vi "dfd_Group Delay Create Specs.vi"(6 "fs [Hz]":dbl=1.0 format="%.2f", 8 "error in (no error)":errorcluster, 10 "freq range":cluster{"f lo":dbl, "f hi":dbl}[](array[cluster]), 11 "filter in":T1={"mSRate_Fs"=1.0, "mSRate_Version"="1.0", "mSRate_Comments"="", "mSRate_OrgCoef"={"type"=enum."Undefined", "gain"=1.0, "coef a (k)"=[], "coef b (v)"=[]}, "mSRate_CurCoef"={"type"=enum."Undefined", "gain"=1.0, "coef a (k)"=[], "coef b (v)"=[]}, "mSRate_Quantized?"=FALSE, "mSRate_QCoef"={"type"=enum."Undefined", "gain"=1.0, "coef a (k)"=[], "coef b (v)"=[]}, "mSRate_QSettings"=[], "mSRate_Order"=0, "mSRate_Scaling"={"mSRate_ScaleByPowerOf2?"=FALSE, "mSRate_ScaleType"=enum."No Norm"}} {"mSRate_QSettings"."source" items=["Coef a/k"=0, "Coef b/v"=7, "Input"=1, "Output"=2, "Multiplicand"=3, "Product"=4, "Sum"=5, "Delay"=6, "Gain"=8]}) -> (0 "error out":errorcluster, 2 "band specs":T7[](array[typedef]) {"subband specs"."weight" format="%.2f"}, 3 "filter out":T1={"mSRate_Fs"=1.0, "mSRate_Version"="1.0", "mSRate_Comments"="", "mSRate_OrgCoef"={"type"=enum."Undefined", "gain"=1.0, "coef a (k)"=[], "coef b (v)"=[]}, "mSRate_CurCoef"={"type"=enum."Undefined", "gain"=1.0, "coef a (k)"=[], "coef b (v)"=[]}, "mSRate_Quantized?"=FALSE, "mSRate_QCoef"={"type"=enum."Undefined", "gain"=1.0, "coef a (k)"=[], "coef b (v)"=[]}, "mSRate_QSettings"=[], "mSRate_Order"=0, "mSRate_Scaling"={"mSRate_ScaleByPowerOf2?"=FALSE, "mSRate_ScaleType"=enum."No Norm"}} {"mSRate_QSettings"."source" items=["Coef a/k"=0, "Coef b/v"=7, "Input"=1, "Output"=2, "Multiplicand"=3, "Product"=4, "Sum"=5, "Delay"=6, "Gain"=8]})   [LabVIEW 2017, in "NI_DigFilter_Design.lvlib"]
uses:
  <vilib>/addons/Digital Filter Design/NI_DigFilter_Design.lvlib
  <vilib>/addons/Digital Filter Design/_GroupDelay.llb/dfd_Group Delay_Band Spec.ctl
  <vilib>/addons/Digital Filter Design/_Objects.llb/DFD Filter Obj.ctl
  <vilib>/addons/Digital Filter Design/_Objects.llb/DFD Filter Coef.ctl
  <vilib>/addons/Digital Filter Design/_Objects.llb/DFD Filter Structure Type Selector.ctl
  <vilib>/addons/Digital Filter Design/_Objects.llb/dfd_Internal Quantization Settings.ctl
  <vilib>/addons/Digital Filter Design/_Objects.llb/dfd_Internal Quantization Srcs.ctl
  <vilib>/addons/Digital Filter Design/_Objects.llb/DFD Coef Norm Type.ctl
  <vilib>/Analysis/1siggen.llb/Ramp Pattern by Samples.vi
  <vilib>/addons/Digital Filter Design/NI_DigFilterLicensed.lvlib
  <vilib>/Analysis/NI_AALBase.lvlib
panel:
  in  "?":T7={"subband specs"=[{"freq"=0.0, "group delay"=1.0, "weight"=1.0}, {"freq"=0.2, "group delay"=1.0, "weight"=1.0}]} {"subband specs"."weight" format="%.2f"}
  # "freq"
  # "group delay"
  # "weight"
  # "freq"
  # "group delay"
  # "weight"
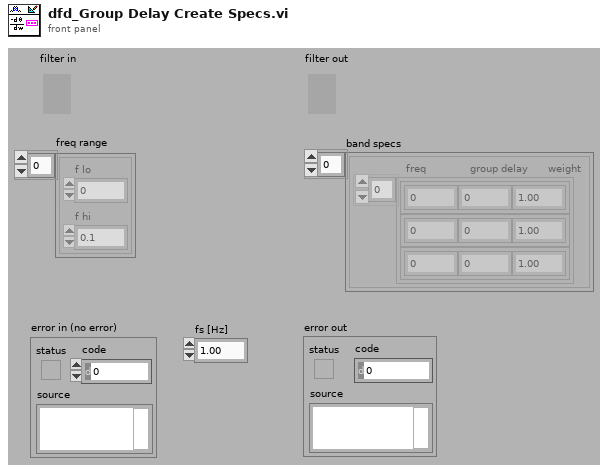
[diagram p1: front panel]
types:
  T1 = typedef "NI_DigFilterLicensed.lvlib/DFD Filter Obj.ctl" = cluster{"mSRate_Fs":dbl, "mSRate_Version":string, "mSRate_Comments":string, "mSRate_OrgCoef":T2, "mSRate_CurCoef":T2, "mSRate_Quantized?":bool, "mSRate_QCoef":T2, "mSRate_QSettings":T4[], "mSRate_Order":i32, "mSRate_Scaling":cluster{"mSRate_ScaleByPowerOf2?":bool, "mSRate_ScaleType":T6}}
  T2 = typedef "NI_DigFilterLicensed.lvlib/DFD Filter Coef.ctl" = cluster{"type":T3, "gain":dbl, "coef a (k)":dbl[], "coef b (v)":dbl[]}
  T3 = typedef "NI_DigFilterLicensed.lvlib/DFD Filter Structure Type Selector.ctl" = enum16{"Undefined", "FIR Direct Form", "FIR Direct Form Transposed", "FIR Symmetric", "FIR Antisymmetric", "IIR Direct Form I", "IIR Direct Form I Transposed", "IIR Direct Form II", "IIR Direct Form II Transposed", "IIR Cascaded Second Order Sections Form I", "IIR Cascaded Second Order Sections Form I Transposed", "IIR Cascaded Second Order Sections Form II", "IIR Cascaded Second Order Sections Form II Transposed", "Lattice Allpass (basic sections)", "Lattice Allpass (one multiplier sections)", "Lattice Allpass (normalized sections)", "Lattice AR (basic sections)", "Lattice AR (one multiplier sections)", "Lattice AR (normalized sections)", "Lattice MA (minimum phase)", "Lattice MA (maximum phase)", "Lattice ARMA (basic sections)", "Lattice ARMA (one multiplier sections)", "Lattice ARMA (normalized sections)"}
  T4 = typedef "NI_DigFilterLicensed.lvlib/dfd_Internal Quantization Settings.ctl" = cluster{"source":T5, "wl":i16, "iwl":i16, "overflow mode":enum16{"Saturation", "Wrap"}, "rounding mode":enum16{"Nearest", "Truncation"}, "signed?":bool}
  T5 = typedef "NI_DigFilterLicensed.lvlib/dfd_Internal Quantization Srcs.ctl" = u16
  T6 = typedef "NI_DigFilterLicensed.lvlib/DFD Coef Norm Type.ctl" = enum16{"No Norm", "Time Domain 1-Norm", "Time Domain 2-Norm", "Time Domain Inf-Norm"}
  T7 = typedef "NI_DigFilterLicensed.lvlib/dfd_Group Delay_Band Spec.ctl" = cluster{"subband specs":cluster{"freq":dbl, "group delay":dbl, "weight":dbl}[]}
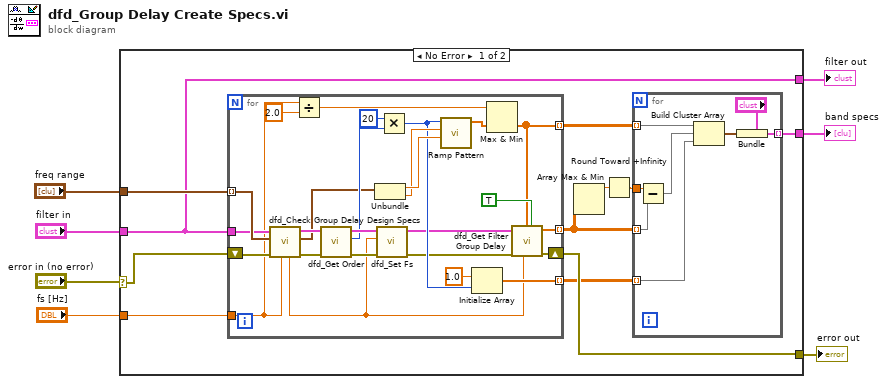
[diagram p0: block diagram]
diagram:
  n1 = case shown="No Error" "error in (no error)" {
    selector: "error in (no error)" -> [w17 w54]
    tunnel: "freq range" -> [w15 _]
    tunnel: "fs [Hz]" -> [w16 _]
    tunnel: "filter in" -> [w13 w53]
    tunnel: [w18 w54] -> w3
    tunnel: [w13 w53] -> w2
    tunnel: [w14 _] -> w1
    frame No Error {
      n2 = for {
        tunnel: w16 -> [w29]
        tunnel: w15 -> [w50] mode=indexing
        tunnel: w13 -> [w49]
        tunnel: [w30] -> w12 mode=indexing
        tunnel: [w47] -> w11 mode=indexing
        tunnel: [w44] -> w10 mode=indexing
        shift-right: [w52] -> w18
        shift-left: w17 -> [w51]
        n3 = call <vilib>:"dfd_Check Group Delay Design Specs.vi"("fs [Hz]"=w29, "error in (no error)"=w51, "freq range"=w50, "filter in"=w49) -> ("error IO"=w35:errorcluster, "dup freq range"=w32:cluster{"f lo":dbl, "f hi":dbl}, "dup filter in"=w33:T1, "dup fs [Hz]"=w34:dbl)  [unwired: 4 out]
        n4 = Divide(x=w29, y=2.0) -> (x/y=w27:dbl)
        n5 = call <vilib>:"dfd_Get Order.vi"("error in (no error)"=w35, "filter in"=w33) -> ("error out"=w41:errorcluster, "order"=w39:i32, "filter out"=w42:T1)  [unwired: 7 out]
        n6 = Unbundle(w32) -> ("f lo"=w46:dbl, "f hi"=w45:dbl)
        n7 = call <vilib>:"dfd_Set Fs.vi"("error in (no error)"=w41, "fs [Hz]"=w34, "filter in"=w42) -> ("error out"=w37:errorcluster, "filter out"=w36:T1)  [unwired: 7 out]
        n8 = Multiply(x=20, y=w39) -> (x*y=w38:i32)
        n9 = call-poly <vilib>:"Ramp Pattern.vi"("start"=w46, "end"=w45, "samples"=w38) -> ("Ramp Pattern"=w31:dbl[])  [unwired: 7 in, 1 out]
        n10 = Initialize Array(1.0 ("element"), w38) -> (w47:dbl[])
        n11 = Max & Min(x=w27, y=w31) -> (min(x,y)=w30:dbl[])  [unwired: 1 out]
        n12 = call <vilib>:"dfd_Get Filter Group Delay.vi"("output option\n(T: FLP)"=TRUE ("output option\n(T: FLP)"), "fs [Hz]"=w34, "freq points [Hz]"=w30, "error in (no error)"=w37, "filter in"=w36) -> ("error out"=w52:errorcluster, "group delay"=w44:dbl[])  [unwired: 5 out]
      }
      n13 = Array Max & Min(array=w10) -> (max value=w9:dbl)  [unwired: 3 out]
      n14 = Round Toward +Infinity(x=w9) -> (ceil(x): smallest int >= x=w8:dbl)
      n15 = for {
        tunnel: [w26] -> w14 mode=indexing
        tunnel: w12 -> [w24] mode=indexing
        tunnel: w11 -> [w22] mode=indexing
        tunnel: w10 -> [w20] mode=indexing
        tunnel: w8 -> [w19]
        n16 = Subtract(x=w19, y=w20) -> (x-y=w25:dbl[])
        n17 = Build Cluster Array(w24, w25, w22) -> (w23:cluster{dbl, dbl, "element":dbl}[])
        n18 = Bundle(cluster="?", "subband specs"=w23) -> (w26:T7)
      }
    }
    frame Error {
    }
  }
  "error out" <- w3
  "band specs" <- w1
  "filter out" <- w2
